vi "Stop AsyncRepeatSum.vi"(8 "error in (no error)":errorcluster, 10 "LVUserEventCallBackRef":refnum<user-event>, 11 "Handle":u64) -> (0 "error out":errorcluster)   [LabVIEW 2016, in "DemoSkeleton.lvlib"]
uses:
  DemoSkeleton.lvlib
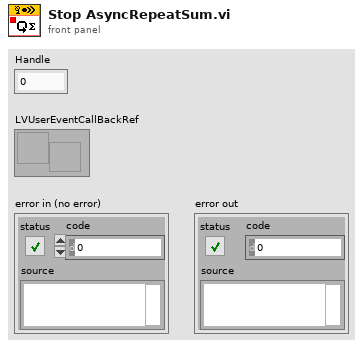
[diagram p1: front panel]
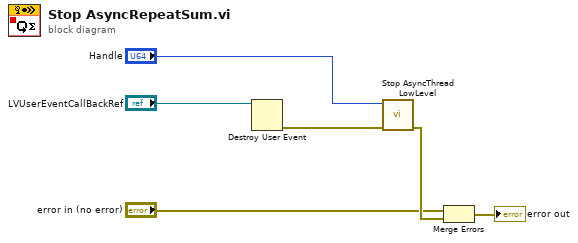
[diagram p0: block diagram]
diagram:
  n1 = Destroy User Event(user event="LVUserEventCallBackRef") -> (error out=w6:errorcluster)  [unwired: 1 in]
  n2 = call "Stop AsyncThread LowLevel.vi"("error in"=w6, "Handle"="Handle") -> ("error out"=w2:errorcluster)  [unwired: 9 in]
  n3 = Merge Errors("error in (no error)", w2) -> (→"error out":errorcluster)
